vi "ConcatenateOntoShortcutMenu.vi"(8 "error in":errorcluster, 9 "menu ref in":refnum<k9>, 11 "node in":refnum<class "RIO Target.lvclass">) -> (0 "error out":errorcluster, 1 "menu ref out":refnum<k9>, 3 "node out":refnum<class "RIO Target.lvclass">)   [LabVIEW 2014, in "RIO Target.lvclass"]
doc: "Allows children to insert menu items without overriding ShortcutMenu.vi entirely. By default, called after Add/Remove."
uses:
  RIO Target.lvclass
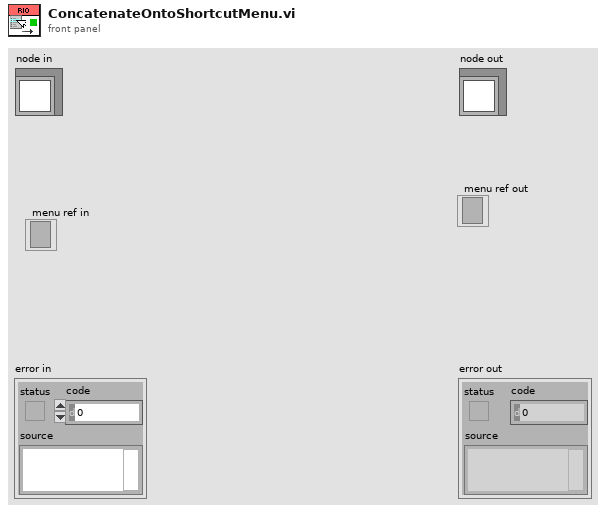
[diagram p1: front panel]
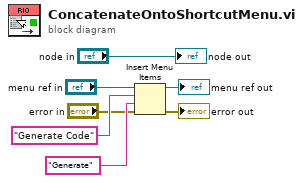
[diagram p0: block diagram]
diagram:
  n1 = Insert Menu Items(6:"error in", 7:"Generate" ("item tags"), 8:"Generate Code", 9:"menu ref in") -> (0:→"error out":errorcluster, 3:→"menu ref out":refnum<k9>)  [unwired: 2 in, 1 out]
  "node out" <- "node in"
